vi "Mod_OFDM_Set_Symbol_Table.vi"(0 "Configuration in":variant=variant("Data Source 0"=variant(cluster{"mode (PN)":enum16{"PN", "pattern", "user"}, "PN sequence order (9)":i32, "base bit pattern (00001111)":enum16{"0", "1", "01", "0011", "00001111"}, "User base bit pattern":i8[]} {"mode (PN)"=enum."PN", "PN sequence order (9)"=9, "base bit pattern (00001111)"=enum."00001111", "User base bit pattern"=[]}), "Data Source 1"=variant(cluster{"mode (PN)":enum16{"PN", "pattern", "user"}, "PN sequence order (9)":i32, "base bit pattern (00001111)":enum16{"0", "1", "01", "0011", "00001111"}, "User base bit pattern":i8[]} {"mode (PN)"=enum."PN", "PN sequence order (9)"=9, "base bit pattern (00001111)"=enum."00001111", "User base bit pattern"=[]}), "Data Source 10"=variant(cluster{"mode (PN)":enum16{"PN", "pattern", "user"}, "PN sequence order (9)":i32, "base bit pattern (00001111)":enum16{"0", "1", "01", "0011", "00001111"}, "User base bit pattern":i8[]} {"mode (PN)"=enum."PN", "PN sequence order (9)"=9, "base bit pattern (00001111)"=enum."00001111", "User base bit pattern"=[]}), "Data Source 11"=variant(cluster{"mode (PN)":enum16{"PN", "pattern", "user"}, "PN sequence order (9)":i32, "base bit pattern (00001111)":enum16{"0", "1", "01", "0011", "00001111"}, "User base bit pattern":i8[]} {"mode (PN)"=enum."PN", "PN sequence order (9)"=9, "base bit pattern (00001111)"=enum."00001111", "User base bit pattern"=[]}), "Data Source 12"=variant(cluster{"mode (PN)":enum16{"PN", "pattern", "user"}, "PN sequence order (9)":i32, "base bit pattern (00001111)":enum16{"0", "1", "01", "0011", "00001111"}, "User base bit pattern":i8[]} {"mode (PN)"=enum."PN", "PN sequence order (9)"=9, "base bit pattern (00001111)"=enum."00001111", "User base bit pattern"=[]}), "Data Source 2"=variant(cluster{"mode (PN)":enum16{"PN", "pattern", "user"}, "PN sequence order (9)":i32, "base bit pattern (00001111)":enum16{"0", "1", "01", "0011", "00001111"}, "User base bit pattern":i8[]} {"mode (PN)"=enum."PN", "PN sequence order (9)"=9, "base bit pattern (00001111)"=enum."00001111", "User base bit pattern"=[]}), "Data Source 3"=variant(cluster{"mode (PN)":enum16{"PN", "pattern", "user"}, "PN sequence order (9)":i32, "base bit pattern (00001111)":enum16{"0", "1", "01", "0011", "00001111"}, "User base bit pattern":i8[]} {"mode (PN)"=enum."PN", "PN sequence order (9)"=9, "base bit pattern (00001111)"=enum."00001111", "User base bit pattern"=[]}), "Data Source 4"=variant(cluster{"mode (PN)":enum16{"PN", "pattern", "user"}, "PN sequence order (9)":i32, "base bit pattern (00001111)":enum16{"0", "1", "01", "0011", "00001111"}, "User base bit pattern":i8[]} {"mode (PN)"=enum."PN", "PN sequence order (9)"=9, "base bit pattern (00001111)"=enum."00001111", "User base bit pattern"=[]}), "Data Source 5"=variant(cluster{"mode (PN)":enum16{"PN", "pattern", "user"}, "PN sequence order (9)":i32, "base bit pattern (00001111)":enum16{"0", "1", "01", "0011", "00001111"}, "User base bit pattern":i8[]} {"mode (PN)"=enum."PN", "PN sequence order (9)"=9, "base bit pattern (00001111)"=enum."00001111", "User base bit pattern"=[]}), "Data Source 6"=variant(cluster{"mode (PN)":enum16{"PN", "pattern", "user"}, "PN sequence order (9)":i32, "base bit pattern (00001111)":enum16{"0", "1", "01", "0011", "00001111"}, "User base bit pattern":i8[]} {"mode (PN)"=enum."PN", "PN sequence order (9)"=9, "base bit pattern (00001111)"=enum."00001111", "User base bit pattern"=[]}), "Data Source 7"=variant(cluster{"mode (PN)":enum16{"PN", "pattern", "user"}, "PN sequence order (9)":i32, "base bit pattern (00001111)":enum16{"0", "1", "01", "0011", "00001111"}, "User base bit pattern":i8[]} {"mode (PN)"=enum."PN", "PN sequence order (9)"=9, "base bit pattern (00001111)"=enum."00001111", "User base bit pattern"=[]}), "Data Source 8"=variant(cluster{"mode (PN)":enum16{"PN", "pattern", "user"}, "PN sequence order (9)":i32, "base bit pattern (00001111)":enum16{"0", "1", "01", "0011", "00001111"}, "User base bit pattern":i8[]} {"mode (PN)"=enum."PN", "PN sequence order (9)"=9, "base bit pattern (00001111)"=enum."00001111", "User base bit pattern"=[]}), "Data Source 9"=variant(cluster{"mode (PN)":enum16{"PN", "pattern", "user"}, "PN sequence order (9)":i32, "base bit pattern (00001111)":enum16{"0", "1", "01", "0011", "00001111"}, "User base bit pattern":i8[]} {"mode (PN)"=enum."PN", "PN sequence order (9)"=9, "base bit pattern (00001111)"=enum."00001111", "User base bit pattern"=[]}), "Modulator 0"=variant(cluster{"M-QAM":enum16{"4", "16", "64", "256", "1024"}, "M-PSK":enum16{"2", "4", "8", "16", "32", "64", "128", "256"}, "Type of Modulation":enum16{"PSK", "QAM"}, "PSK":cluster{"differential PSK":enum16{"disable", "enable"}, "PSK type":u16}} {"M-QAM"=enum."4", "M-PSK"=enum."2", "Type of Modulation"=enum."PSK", "PSK"={"differential PSK"=enum."disable", "PSK type"=0}}), "Modulator 1"=variant(cluster{"M-QAM":enum16{"4", "16", "64", "256", "1024"}, "M-PSK":enum16{"2", "4", "8", "16", "32", "64", "128", "256"}, "Type of Modulation":enum16{"PSK", "QAM"}, "PSK":cluster{"differential PSK":enum16{"disable", "enable"}, "PSK type":u16}} {"M-QAM"=enum."4", "M-PSK"=enum."2", "Type of Modulation"=enum."PSK", "PSK"={"differential PSK"=enum."disable", "PSK type"=0}}), "Modulator 10"=variant(cluster{"M-QAM":enum16{"4", "16", "64", "256", "1024"}, "M-PSK":enum16{"2", "4", "8", "16", "32", "64", "128", "256"}, "Type of Modulation":enum16{"PSK", "QAM"}, "PSK":cluster{"differential PSK":enum16{"disable", "enable"}, "PSK type":u16}} {"M-QAM"=enum."4", "M-PSK"=enum."2", "Type of Modulation"=enum."PSK", "PSK"={"differential PSK"=enum."disable", "PSK type"=0}}), "Modulator 11"=variant(cluster{"M-QAM":enum16{"4", "16", "64", "256", "1024"}, "M-PSK":enum16{"2", "4", "8", "16", "32", "64", "128", "256"}, "Type of Modulation":enum16{"PSK", "QAM"}, "PSK":cluster{"differential PSK":enum16{"disable", "enable"}, "PSK type":u16}} {"M-QAM"=enum."4", "M-PSK"=enum."2", "Type of Modulation"=enum."PSK", "PSK"={"differential PSK"=enum."disable", "PSK type"=0}}), "Modulator 12"=variant(cluster{"M-QAM":enum16{"4", "16", "64", "256", "1024"}, "M-PSK":enum16{"2", "4", "8", "16", "32", "64", "128", "256"}, "Type of Modulation":enum16{"PSK", "QAM"}, "PSK":cluster{"differential PSK":enum16{"disable", "enable"}, "PSK type":u16}} {"M-QAM"=enum."4", "M-PSK"=enum."2", "Type of Modulation"=enum."PSK", "PSK"={"differential PSK"=enum."disable", "PSK type"=0}}), "Modulator 2"=variant(cluster{"M-QAM":enum16{"4", "16", "64", "256", "1024"}, "M-PSK":enum16{"2", "4", "8", "16", "32", "64", "128", "256"}, "Type of Modulation":enum16{"PSK", "QAM"}, "PSK":cluster{"differential PSK":enum16{"disable", "enable"}, "PSK type":u16}} {"M-QAM"=enum."4", "M-PSK"=enum."2", "Type of Modulation"=enum."PSK", "PSK"={"differential PSK"=enum."disable", "PSK type"=0}}), "Modulator 3"=variant(cluster{"M-QAM":enum16{"4", "16", "64", "256", "1024"}, "M-PSK":enum16{"2", "4", "8", "16", "32", "64", "128", "256"}, "Type of Modulation":enum16{"PSK", "QAM"}, "PSK":cluster{"differential PSK":enum16{"disable", "enable"}, "PSK type":u16}} {"M-QAM"=enum."4", "M-PSK"=enum."2", "Type of Modulation"=enum."PSK", "PSK"={"differential PSK"=enum."disable", "PSK type"=0}}), "Modulator 4"=variant(cluster{"M-QAM":enum16{"4", "16", "64", "256", "1024"}, "M-PSK":enum16{"2", "4", "8", "16", "32", "64", "128", "256"}, "Type of Modulation":enum16{"PSK", "QAM"}, "PSK":cluster{"differential PSK":enum16{"disable", "enable"}, "PSK type":u16}} {"M-QAM"=enum."4", "M-PSK"=enum."2", "Type of Modulation"=enum."PSK", "PSK"={"differential PSK"=enum."disable", "PSK type"=0}}), "Modulator 5"=variant(cluster{"M-QAM":enum16{"4", "16", "64", "256", "1024"}, "M-PSK":enum16{"2", "4", "8", "16", "32", "64", "128", "256"}, "Type of Modulation":enum16{"PSK", "QAM"}, "PSK":cluster{"differential PSK":enum16{"disable", "enable"}, "PSK type":u16}} {"M-QAM"=enum."4", "M-PSK"=enum."2", "Type of Modulation"=enum."PSK", "PSK"={"differential PSK"=enum."disable", "PSK type"=0}}), "Modulator 6"=variant(cluster{"M-QAM":enum16{"4", "16", "64", "256", "1024"}, "M-PSK":enum16{"2", "4", "8", "16", "32", "64", "128", "256"}, "Type of Modulation":enum16{"PSK", "QAM"}, "PSK":cluster{"differential PSK":enum16{"disable", "enable"}, "PSK type":u16}} {"M-QAM"=enum."4", "M-PSK"=enum."2", "Type of Modulation"=enum."PSK", "PSK"={"differential PSK"=enum."disable", "PSK type"=0}}), "Modulator 7"=variant(cluster{"M-QAM":enum16{"4", "16", "64", "256", "1024"}, "M-PSK":enum16{"2", "4", "8", "16", "32", "64", "128", "256"}, "Type of Modulation":enum16{"PSK", "QAM"}, "PSK":cluster{"differential PSK":enum16{"disable", "enable"}, "PSK type":u16}} {"M-QAM"=enum."4", "M-PSK"=enum."2", "Type of Modulation"=enum."PSK", "PSK"={"differential PSK"=enum."disable", "PSK type"=0}}), "Modulator 8"=variant(cluster{"M-QAM":enum16{"4", "16", "64", "256", "1024"}, "M-PSK":enum16{"2", "4", "8", "16", "32", "64", "128", "256"}, "Type of Modulation":enum16{"PSK", "QAM"}, "PSK":cluster{"differential PSK":enum16{"disable", "enable"}, "PSK type":u16}} {"M-QAM"=enum."4", "M-PSK"=enum."2", "Type of Modulation"=enum."PSK", "PSK"={"differential PSK"=enum."disable", "PSK type"=0}}), "Modulator 9"=variant(cluster{"M-QAM":enum16{"4", "16", "64", "256", "1024"}, "M-PSK":enum16{"2", "4", "8", "16", "32", "64", "128", "256"}, "Type of Modulation":enum16{"PSK", "QAM"}, "PSK":cluster{"differential PSK":enum16{"disable", "enable"}, "PSK type":u16}} {"M-QAM"=enum."4", "M-PSK"=enum."2", "Type of Modulation"=enum."PSK", "PSK"={"differential PSK"=enum."disable", "PSK type"=0}}), "Sub Carrier 0"=variant(cluster{"Data Source Control":cluster{"mode (PN)":enum16{"PN", "pattern", "user"}, "PN sequence order (9)":i32, "base bit pattern (00001111)":enum16{"0", "1", "01", "0011", "00001111"}, "User base bit pattern":i8[]}, "Modulator Control":cluster{"M-QAM":enum16{"4", "16", "64", "256", "1024"}, "M-PSK":enum16{"2", "4", "8", "16", "32", "64", "128", "256"}, "Type of Modulation":enum16{"PSK", "QAM"}, "PSK":cluster{"differential PSK":enum16{"disable", "enable"}, "PSK type":u16}}, "Sub Carrier":bool, string, string} {"Data Source Control"={"mode (PN)"=enum."PN", "PN sequence order (9)"=9, "base bit pattern (00001111)"=enum."00001111", "User base bit pattern"=[]}, "Modulator Control"={"M-QAM"=enum."4", "M-PSK"=enum."2", "Type of Modulation"=enum."PSK", "PSK"={"differential PSK"=enum."disable", "PSK type"=0}}, "Sub Carrier"=TRUE, "Data Source 0", "Modulator 3"})), 7 "Current OFDM \nSymbol NAME":string, 11 "error in":errorcluster, 12 "Symbol Pool":u16(ring), 13 "Configure/\nRetrieve":bool) -> (2 "OFDM Parameters":T1, 4 "Configuration out":variant, 8 "Symbol Table":string[][](array[string]), 10 "Current OFDM Symbol Name(O/P)":string, 15 "error out":errorcluster)   [LabVIEW 2010]
uses:
  Controls(Type_DEf)/Configure Pulse Shaping.ctl
  Controls(Type_DEf)/Pool of Modulator Control.ctl
  Controls(Type_DEf)/Pool of Data Source Control.ctl
  Controls(Type_DEf)/Attribute Names.ctl
  MOD_OFDM_Get_Attr.vi
  Mod_OFDM_Set_Ofdm_Parameters.vi
panel:
  in  "Attribute Data Types":T6={"Pulse Shaping"={"System Filter"={"TX Filter"=enum."none", "Alpha"=0.0, "filter length"=0}, "Modulation system parameters"={"samples per symbol (16)"=0}, "symbol rate (Hz)"=0.0}, "FRAME Table"=[], "OFDM Frame"=[], "Sub Carrier Selection"={"Sub Carrier Selection"=[], "OFDM Parameters"={"# of Sub Carrier"=64, "Length Of Cylic Prefix"=16}}, "Symbol Table"=[], "Symbol Pool"=[], "Pool of Modulators"=[], "Pool of Data Sources"=[], "Atribute Names"={"Data Source Pool"="Data Source Pool ", "Modulator Source Pool"="Modulator Source Pool ", "OFDM SYMBOL POOL"="OFDM SYMBOL POOL", "Symbol Table"="Symbol Table", "Sub Carrier Selection"="Sub Carrier Selection", "OFDM Frame"="OFDM Frame", "FRAME Table"="FRAME Table", "Pulse Shaping"="Pulse Shaping"}} {"Pool of Data Sources"."Register Initial State" format="%08x"; "Pulse Shaping"."symbol rate (Hz)" min=1.0 step=1.0 format="%.2p"; "Pulse Shaping"."Modulation system parameters"."samples per symbol (16)" step=2; "Pulse Shaping"."System Filter"."Alpha" min=0.0 max=1.0 step=0.05 format="%.2f"}
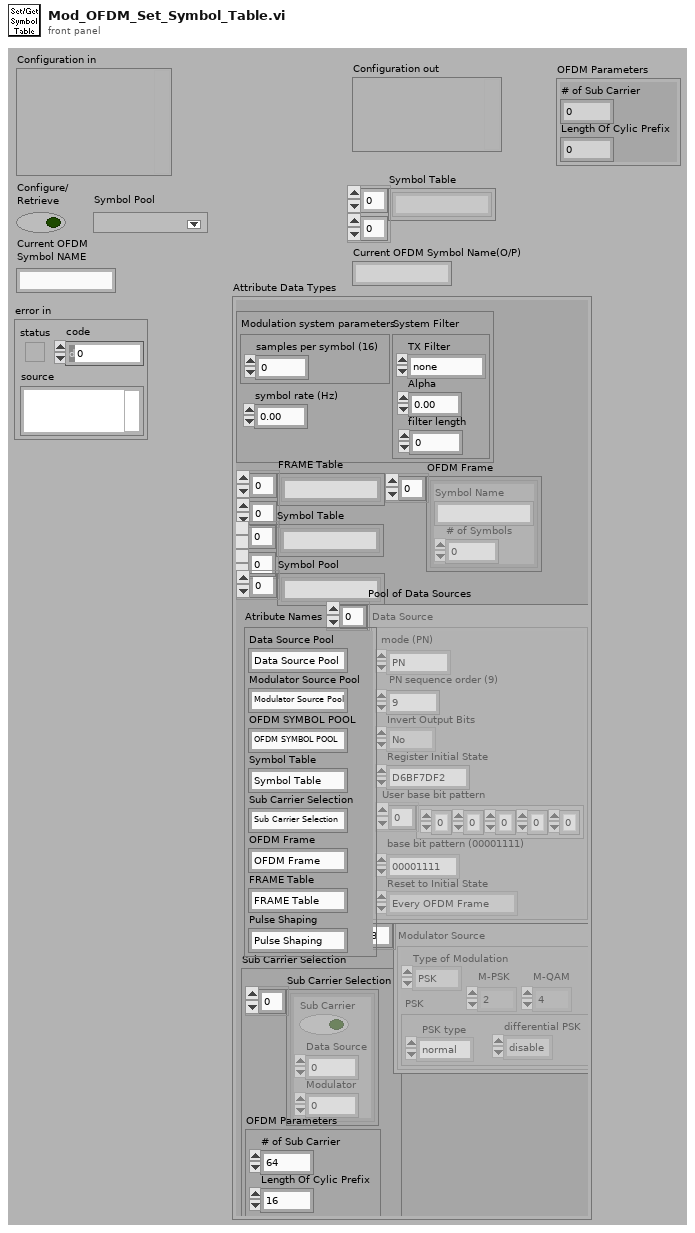
[diagram p1: front panel]
types:
  T1 = cluster{"# of Sub Carrier":i32, "Length Of Cylic Prefix":i32}
  T2 = typedef "Configure Pulse Shaping.ctl" = cluster{"System Filter":cluster{"TX Filter":enum16{"none", "Raised Cosine", "Root Raised Cos"}, "Alpha":dbl, "filter length":i32}, "Modulation system parameters":cluster{"samples per symbol (16)":u32}, "symbol rate (Hz)":dbl}
  T3 = typedef "Pool of Modulator Control.ctl" = cluster{"M-QAM":enum16{"4", "16", "64", "256"}, "M-PSK":enum16{"2", "4", "8", "16", "32", "64", "128", "256"}, "Type of Modulation":enum16{"PSK", "QAM"}, " PSK":cluster{"differential PSK":enum16{"disable", "enable"}, "PSK type":enum16{"normal", "shifted", "offset"}}}[]
  T4 = typedef "Pool of Data Source Control.ctl" = cluster{"mode (PN)":enum16{"PN", "pattern", "user"}, "PN sequence order (9)":i32, "Invert Output Bits":enum16{"No", "Yes"}, "Register Initial State ":u32, "User base bit pattern":i8[], "base bit pattern (00001111)":enum16{"0", "1", "01", "0011", "00001111"}, "Reset to Initial State":enum16{"Every OFDM Frame", "Every OFDM Symbol", "Every Sub Carrier"}}[]
  T5 = typedef "Attribute Names.ctl" = cluster{"Data Source Pool":string, "Modulator Source Pool":string, "OFDM SYMBOL POOL":string, "Symbol Table":string, "Sub Carrier Selection":string, "OFDM Frame":string, "FRAME Table":string, "Pulse Shaping":string}
  T6 = cluster{"Pulse Shaping":T2, "FRAME Table":string[][], "OFDM Frame":cluster{"Symbol Name":string, "# of Symbols":i32}[], "Sub Carrier Selection":cluster{"Sub Carrier Selection":cluster{"Sub Carrier":bool, "Data Source":u16, "Modulator":u16}[], "OFDM Parameters":cluster{"# of Sub Carrier":i32, "Length Of Cylic Prefix":i32}}, "Symbol Table":string[][], "Symbol Pool":string[], "Pool of Modulators":T3, "Pool of Data Sources":T4, "Atribute Names":T5}
  T7 = cluster{"Sub Carrier Selection":cluster{"Sub Carrier":bool, "Data Source":u16, "Modulator":u16}[], "OFDM Parameters":cluster{"# of Sub Carrier":i32, "Length Of Cylic Prefix":i32}}
  T8 = cluster{"Sub Carrier":bool, "Data Source":u16, "Modulator":u16}[]
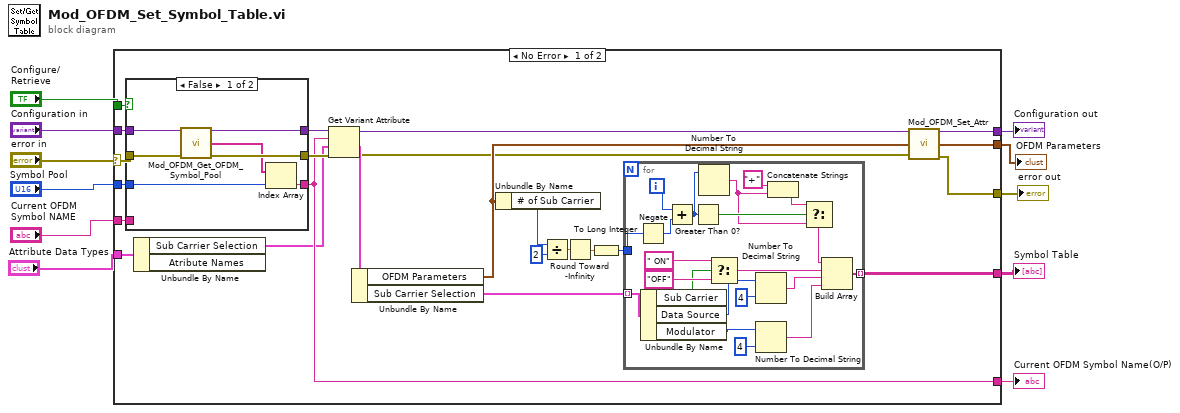
[diagram p0: block diagram]
diagram:
  n1 = case shown="No Error" "error in" {
    selector: "error in" -> [w28 w66]
    tunnel: "Symbol Pool" -> [w34 _]
    tunnel: "Current OFDM \nSymbol NAME" -> [w32 _]
    tunnel: [w31 _] -> w9
    tunnel: "Configure/\nRetrieve" -> [w30 _]
    tunnel: "Configuration in" -> [w29 _]
    tunnel: [w22 _] -> w6
    tunnel: [w23 w66] -> w4
    tunnel: "Attribute Data Types" -> [w26 _]
    tunnel: [w24 _] -> w2
    tunnel: [w19 _] -> w1
    frame No Error {
      n2 = case shown="False" w30 {
        tunnel: w29 -> [w39 w42]
        tunnel: w34 -> [w41 _]
        tunnel: w28 -> [w38 w43]
        tunnel: [w37 w43] -> w33
        tunnel: w32 -> [_ w44]
        tunnel: [w40 w44] -> w31
        tunnel: [w35 w42] -> w25
        frame False {
          n3 = call-poly "Mod_OFDM_Get_OFDM_Symbol_Pool.vi"("Configuration in"=w39, "error in"=w38) -> ("Configuration out"=w35:variant, "Symbol Pool"=w36:string[], "error out"=w37:errorcluster)  [unwired: 8 in, 3 out]
          n4 = Index Array(array=w36, index=w41) -> (element=w40:string)
        }
        frame True {
        }
      }
      n5 = Unbundle By Name(w26) -> ("Sub Carrier Selection"=w21:T7)  [unwired: 1 out]
      n6 = Get Variant Attribute(Variant=w25, name=w31, default value (empty Variant)=w21, error in=w33) -> (duplicate Variant=w13:variant, value=w27:T7, error out=w12:errorcluster)  [unwired: 1 out]
      n7 = Unbundle By Name(w27) -> ("OFDM Parameters"=w19:T1, "Sub Carrier Selection"=w20:T8)
      n8 = Unbundle By Name(w19) -> ("# of Sub Carrier"=w18:i32)
      n9 = Divide(x=w18, y=2) -> (x/y=w16:dbl)
      n10 = Round Toward -Infinity(1:w16) -> (0:w15:dbl)
      n11 = To Long Integer(number=w15) -> (32bit integer=w14:i32)
      n12 = for {
        tunnel: w20 -> [w62] mode=indexing
        tunnel: [w57] -> w24 mode=indexing
        tunnel: w14 -> [w48]
        i -> [w55]
        n13 = Negate(x=w48) -> (-x=w47:i32)
        n14 = Unbundle By Name(w62) -> ("Sub Carrier"=w56:bool, "Data Source"=w58:u16, "Modulator"=w61:u16)
        n15 = Add(x=w55, y=w47) -> (x+y=w54:i32)
        n16 = Greater Than 0?(x=w54) -> (x > 0?=w53:bool)
        n17 = Number To Decimal String(number=w54) -> (decimal integer string=w49:string)  [unwired: 1 in]
        n18 = Select(t=" ON", s=w56, f="OFF") -> (s? t:f=w63:string)
        n19 = Number To Decimal String(number=w58, width (-)=i16 4) -> (decimal integer string=w60:string)
        n20 = Number To Decimal String(number=w61, width (-)=i16 4) -> (decimal integer string=w59:string)
        n21 = Concatenate Strings("+", w49) -> (w52:string)
        n22 = Select(t=w52, s=w53, f=w49) -> (s? t:f=w51:string)
        n23 = Build Array(w51, w63, w60, w59) -> (w57:string[])
      }
      n24 = call-poly "Mod_OFDM_Set_Attr.vi"("Configuration in"=w13, "OFDM Parameters"=w19, "error in"=w12) -> ("Configuration out"=w22:variant, "error out"=w23:errorcluster)  [unwired: 11 in]
    }
    frame Error {
    }
  }
  "error out" <- w4
  "Configuration out" <- w6
  "Current OFDM Symbol Name(O/P)" <- w9
  "Symbol Table" <- w2
  "OFDM Parameters" <- w1
